vi "FITS_Test_Record.vi"() -> ()   [LabVIEW 2016]
panel:
  in  "Keyword Value":string="12:00:01"
  in  "Keyword Name":string="TIME    "
  out "Color Table 2":u32[](array[numeric])=[0, 65793, 131586, 197379, 263172, 328965, 394758, 460551, 526344, 592137, 657930, 723723, 789516, 855309, 921102, 986895, 1052688, 1118481, 1184274, 1250067, 1315860, 1381653, 1447446, 1513239, 1579032, 1644825, 1710618, 1776411, 1842204, 1907997, 1973790, 2039583, 2105376, 2171169, 2236962, 2302755, 2368548, 2434341, 2500134, 2565927, 2631720, 2697513, 2763306, 2829099, 2894892, 2960685, 3026478, 3092271, 3158064, 3223857, 3289650, 3355443, 3421236, 3487029, 3552822, 3618615, 3684408, 3750201, 3815994, 3881787, 3947580, 4013373, 4079166, 4144959, 4210752, 4276545, 4342338, 4408131, 4473924, 4539717, 4605510, 4671303, 4737096, 4802889, 4868682, 4934475, 5000268, 5066061, 5131854, 5197647, 5263440, 5329233, 5395026, 5460819, 5526612, 5592405, 5658198, 5723991, 5789784, 5855577, 5921370, 5987163, 6052956, 6118749, 6184542, 6250335, 6316128, 6381921, 6447714, 6513507, 6579300, 6645093, 6710886, 6776679, 6842472, 6908265, 6974058, 7039851, 7105644, 7171437, 7237230, 7303023, 7368816, 7434609, 7500402, 7566195, 7631988, 7697781, 7763574, 7829367, 7895160, 7960953, 8026746, 8092539, 8158332, 8224125, 8289918, 8355711, 8421504, 8487297, 8553090, 8618883, 8684676, 8750469, 8816262, 8882055, 8947848, 9013641, 9079434, 9145227, 9211020, 9276813, 9342606, 9408399, 9474192, 9539985, 9605778, 9671571, 9737364, 9803157, 9868950, 9934743, 10000536, 10066329, 10132122, 10197915, 10263708, 10329501, 10395294, 10461087, 10526880, 10592673, 10658466, 10724259, 10790052, 10855845, 10921638, 10987431, 11053224, 11119017, 11184810, 11250603, 11316396, 11382189, 11447982, 11513775, 11579568, 11645361, 11711154, 11776947, 11842740, 11908533, 11974326, 12040119, 12105912, 12171705, 12237498, 12303291, 12369084, 12434877, 12500670, 12566463, 12632256, 12698049, 12763842, 12829635, 12895428, 12961221, 13027014, 13092807, 13158600, 13224393, 13290186, 13355979, 13421772, 13487565, 13553358, 13619151, 13684944, 13750737, 13816530, 13882323, 13948116, 14013909, 14079702, 14145495, 14211288, 14277081, 14342874, 14408667, 14474460, 14540253, 14606046, 14671839, 14737632, 14803425, 14869218, 14935011, 15000804, 15066597, 15132390, 15198183, 15263976, 15329769, 15395562, 15461355, 15527148, 15592941, 15658734, 15724527, 15790320, 15856113, 15921906, 15987699, 16053492, 16119285, 16185078, 16250871, 16316664, 16382457, 16448250, 16514043, 16579836, 16645629, 16711422, 16777215] format="%.0x"
  out "Color Table":u32[](array[colorbox])=[0, 65793, 131586, 197379, 263172, 328965, 394758, 460551, 526344, 592137, 657930, 723723, 789516, 855309, 921102, 986895, 1052688, 1118481, 1184274, 1250067, 1315860, 1381653, 1447446, 1513239, 1579032, 1644825, 1710618, 1776411, 1842204, 1907997, 1973790, 2039583, 2105376, 2171169, 2236962, 2302755, 2368548, 2434341, 2500134, 2565927, 2631720, 2697513, 2763306, 2829099, 2894892, 2960685, 3026478, 3092271, 3158064, 3223857, 3289650, 3355443, 3421236, 3487029, 3552822, 3618615, 3684408, 3750201, 3815994, 3881787, 3947580, 4013373, 4079166, 4144959, 4210752, 4276545, 4342338, 4408131, 4473924, 4539717, 4605510, 4671303, 4737096, 4802889, 4868682, 4934475, 5000268, 5066061, 5131854, 5197647, 5263440, 5329233, 5395026, 5460819, 5526612, 5592405, 5658198, 5723991, 5789784, 5855577, 5921370, 5987163, 6052956, 6118749, 6184542, 6250335, 6316128, 6381921, 6447714, 6513507, 6579300, 6645093, 6710886, 6776679, 6842472, 6908265, 6974058, 7039851, 7105644, 7171437, 7237230, 7303023, 7368816, 7434609, 7500402, 7566195, 7631988, 7697781, 7763574, 7829367, 7895160, 7960953, 8026746, 8092539, 8158332, 8224125, 8289918, 8355711, 8421504, 8487297, 8553090, 8618883, 8684676, 8750469, 8816262, 8882055, 8947848, 9013641, 9079434, 9145227, 9211020, 9276813, 9342606, 9408399, 9474192, 9539985, 9605778, 9671571, 9737364, 9803157, 9868950, 9934743, 10000536, 10066329, 10132122, 10197915, 10263708, 10329501, 10395294, 10461087, 10526880, 10592673, 10658466, 10724259, 10790052, 10855845, 10921638, 10987431, 11053224, 11119017, 11184810, 11250603, 11316396, 11382189, 11447982, 11513775, 11579568, 11645361, 11711154, 11776947, 11842740, 11908533, 11974326, 12040119, 12105912, 12171705, 12237498, 12303291, 12369084, 12434877, 12500670, 12566463, 12632256, 12698049, 12763842, 12829635, 12895428, 12961221, 13027014, 13092807, 13158600, 13224393, 13290186, 13355979, 13421772, 13487565, 13553358, 13619151, 13684944, 13750737, 13816530, 13882323, 13948116, 14013909, 14079702, 14145495, 14211288, 14277081, 14342874, 14408667, 14474460, 14540253, 14606046, 14671839, 14737632, 14803425, 14869218, 14935011, 15000804, 15066597, 15132390, 15198183, 15263976, 15329769, 15395562, 15461355, 15527148, 15592941, 15658734, 15724527, 15790320, 15856113, 15921906, 15987699, 16053492, 16119285, 16185078, 16250871, 16316664, 16382457, 16448250, 16514043, 16579836, 16645629, 16711422, 16777215]
  in  "Intensity Graph":sgl[][](graph)=array128x128[16384 elements]
  out "error out":errorcluster
  in  "Path":path=path "/home/ao/RTsoft/LV86Modules/FITS-3.0/test/record_test.fits"
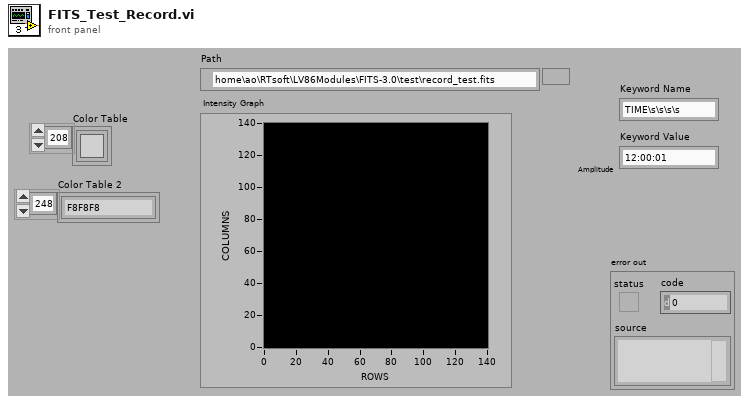
[diagram p1: front panel]
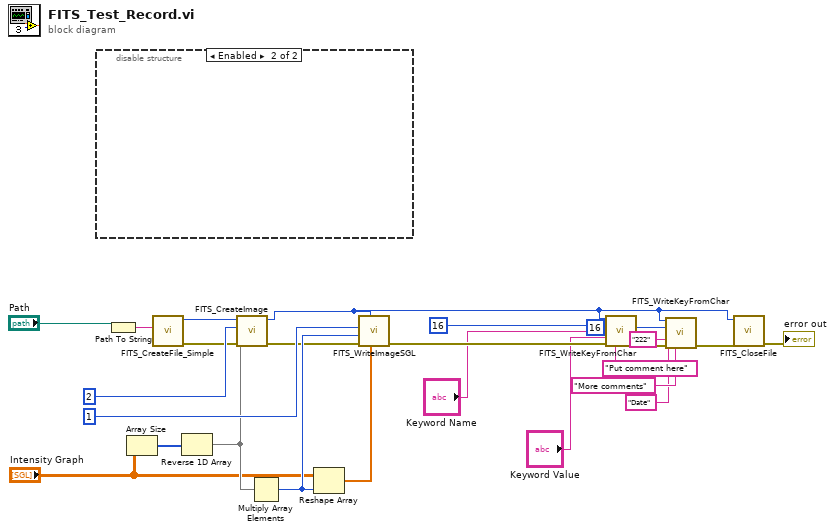
[diagram p0: block diagram]
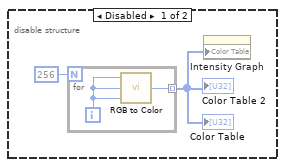
[diagram p2: hidden frame]
diagram:
  n1 = disable-structure shown="Enabled" {
    frame Disabled {
      n2 = for {
        N: 256 -> [_]
        tunnel: [w28] -> w26 mode=indexing
        i -> [w29]
        n3 = call <vilib>:"RGB to Color.vi"("B"=w29, "G"=w29, "R"=w29) -> ("Color"=w28:u32)
      }
      "Color Table" <- w26
      "Color Table 2" <- w26
      n4 = property on="Intensity Graph" class="IntGraph (strict)"("Color Table"=w26) -> ()  [unwired: 2 in, 2 out]
    }
    frame Enabled {
    }
  }
  n5 = Path To String(path="Path") -> (string=w25:string)
  n6 = Array Size(array="Intensity Graph") -> (size(s)=w18:i32[])
  n7 = call "FITS_CreateFile_Simple.vi"("filename"=w25) -> ("error out"=w23:errorcluster, "fd"=w8:u64)  [unwired: 1 in, 8 out]
  n8 = Reverse 1D Array(array=w18) -> (reversed array=w17:i32[])
  n9 = call "FITS_CreateImage.vi"("error in"=w23, "naxes"=w17, "naxis"=2, "ref in"=w8) -> ("error out"=w20:errorcluster, "ref out"=w2:u64)  [unwired: 1 in, 5 out]
  n10 = Multiply Array Elements(1:w17) -> (0:w21:i32)
  n11 = Reshape Array("Intensity Graph", w21) -> (w19:sgl[])
  n12 = call "FITS_WriteImageSGL.vi"("Array"=w19, "ref"=w2, "error in"=w20, "nelem"=w21, "firstel"=1) -> ("error out"=w13:errorcluster)  [unwired: 5 in, 1 out]
  n13 = call "FITS_WriteKeyFromChar.vi"("ref"=w2, "datatype"=16, "keyname"="Keyword Name", "value"="Keyword Value", "error in (no error)"=w13, "comment"="Put comment here") -> ("error out"=w7:errorcluster)  [unwired: 5 in, 4 out]
  n14 = call "FITS_WriteKeyFromChar.vi"("ref"=w2, "datatype"=16, "keyname"="Date", "value"="222", "error in (no error)"=w7, "comment"="More comments") -> ("error out"=w6:errorcluster)  [unwired: 5 in, 4 out]
  n15 = call "FITS_CloseFile.vi"("error in"=w6, "ref in"=w2) -> ("error out"=→"error out":errorcluster)  [unwired: 1 in, 8 out]
